vi "Find All Zeroes Inner Part.vi"(3 "accuracy":dbl=1e-08 format="%.2e", 4 "algorithm":u16, 5 "formula":string, 6 "X and Y values":cluster{"X Values":dbl[], "Y Values":dbl[]} {"Y Values" format="%.2f"; "X Values" format="%.2f"}) -> (0 "error":i32, 1 "f(Zeroes)":dbl[](array[numeric]) format="%.2f", 2 "Zeroes":dbl[](array[numeric]) format="%.2f")   [LabVIEW 2018, in "NI_Gmath.lvlib"]
uses:
  NI_Gmath.lvlib
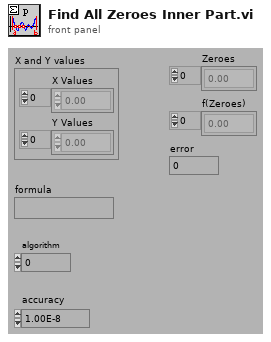
[diagram p1: front panel]
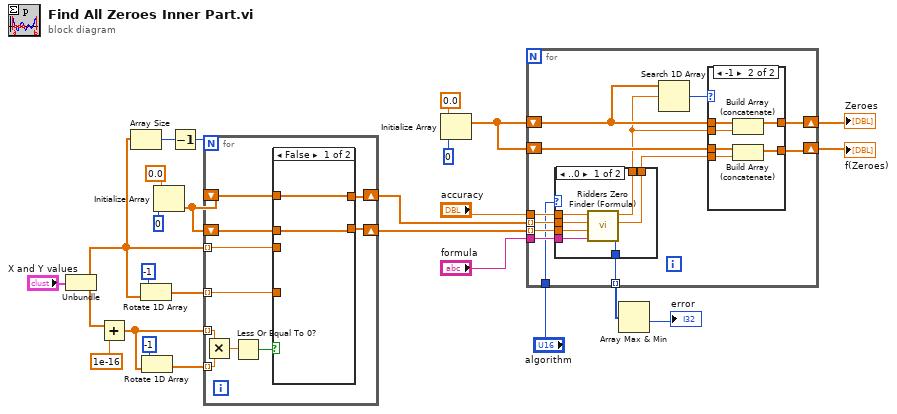
[diagram p0: block diagram]
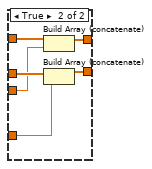
[diagram p2: hidden frame]
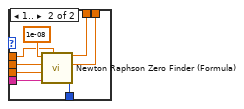
[diagram p4: hidden frame]
diagram:
  n1 = Unbundle("X and Y values") -> ("X Values"=w12:dbl[], "Y Values"=w6:dbl[])
  n2 = Add(x=w6, y=1e-16) -> (x+y=w8:dbl[])
  n3 = Array Size(array=w12) -> (size(s)=w2:i32)
  n4 = Rotate 1D Array(1:w12, 2:-1) -> (0:w14:dbl[])
  n5 = Rotate 1D Array(1:w8, 2:-1) -> (0:w5:dbl[])
  n6 = Initialize Array(0.0, 0) -> (w11:dbl[])
  n7 = Decrement(x=w2) -> (x-1=w3:i32)
  n8 = for {
    N: w3 -> [_]
    tunnel: w8 -> [w36] mode=indexing
    tunnel: w5 -> [w35] mode=indexing
    shift-right: [w31] -> w1
    shift-left: w11 -> [w32]
    shift-right: [w29] -> w20
    shift-left: w11 -> [w30]
    tunnel: w12 -> [w28] mode=indexing
    tunnel: w14 -> [w27] mode=indexing
    n9 = Multiply(x=w36, y=w35) -> (x*y=w34:dbl)
    n10 = Less Or Equal To 0?(x=w34) -> (x <= 0?=w33:bool)
    n11 = case shown="False" w33 {
      tunnel: w32 -> [w38 w44]
      tunnel: [w38 w43] -> w31
      tunnel: w30 -> [w37 w42]
      tunnel: [w37 w41] -> w29
      tunnel: w28 -> [_ w40]
      tunnel: w27 -> [_ w39]
      frame False {
      }
      frame True {
        n12 = Build Array (concatenate)(w44, w40) -> (w43:dbl[])
        n13 = Build Array (concatenate)(w42, w39) -> (w41:dbl[])
      }
    }
  }
  n14 = Initialize Array(0.0, 0) -> (w19:dbl[])
  n15 = for {
    tunnel: w1 -> [w53] mode=indexing
    tunnel: w20 -> [w52] mode=indexing
    tunnel: "accuracy" -> [w50]
    tunnel: "formula" -> [w51]
    shift-right: [w55] -> w24
    shift-left: w19 -> [w47]
    shift-right: [w56] -> w25
    shift-left: w19 -> [w57]
    tunnel: "algorithm" -> [w49]
    tunnel: [w48] -> w23 mode=indexing
    n16 = case shown="..0" w49 {
      tunnel: w50 -> [w72 w79]
      tunnel: w51 -> [w69 w76]
      tunnel: w52 -> [w70 w77]
      tunnel: w53 -> [w71 w78]
      tunnel: [w67 w74] -> w54
      tunnel: [w68 w75] -> w46
      tunnel: [w66 w73] -> w48
      frame ..0 {
        n17 = call "Ridders Zero Finder (Formula).vi"("formula"=w69, "end"=w70, "start"=w71, "accuracy"=w72) -> ("error"=w66:i32, "f(zero)"=w67:dbl, "zero"=w68:dbl)  [unwired: 5 out]
      }
      frame 1.. {
        n18 = call "Newton Raphson Zero Finder (Formula).vi"("accuracy"=w79, "formula"=w76, "end"=w77, "start"=w78, "h"=1e-08) -> ("error"=w73:i32, "f(zero)"=w74:dbl, "zero"=w75:dbl)  [unwired: 4 out]
      }
    }
    n19 = Search 1D Array(1D array=w47, element=w46) -> (index of element=w45:i32)  [unwired: 1 in]
    n20 = case shown="-1" w45 {
      tunnel: w57 -> [w58 w65]
      tunnel: [w58 w64] -> w56
      tunnel: [w59 w63] -> w55
      tunnel: w54 -> [_ w62]
      tunnel: w47 -> [w59 w61]
      tunnel: w46 -> [_ w60]
      frame 0, Default {
      }
      frame -1 {
        n21 = Build Array (concatenate)(w61, w60) -> (w63:dbl[])
        n22 = Build Array (concatenate)(w65, w62) -> (w64:dbl[])
      }
    }
  }
  "f(Zeroes)" <- w25
  "Zeroes" <- w24
  n23 = Array Max & Min(array=w23) -> (min value=→"error":i32)  [unwired: 3 out]
